vi "Is Created Queue.vi"(10 "Created Queue Alias":string, 11 "Queue in":refnum<class "Queue.lvclass">) -> (2 "Is Created Queue?":bool, 3 "Queue out":refnum<class "Queue.lvclass">)   [LabVIEW 2021, in "jettl.lvlib" / "Queue.lvclass"]
uses:
  Queue.lvclass
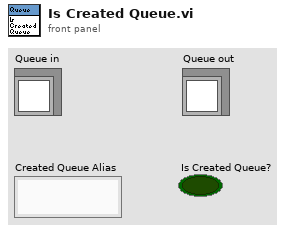
[diagram p1: front panel]
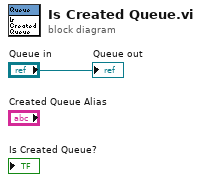
[diagram p0: block diagram]
diagram:
  "Queue out" <- "Queue in"
